vi "PWM Servo RT.vi"() -> ()   [LabVIEW 2012]
uses:
  <vilib>/FPGAPlugInAG/cRIO-9074/niLvFpga_Open_cRIO-9074.vi
  <vilib>/rvi/interface/common/dynamic/niFpgaDynamicAddResources.vi
  <vilib>/Utility/error.llb/Error Cluster From Error Code.vi
  <vilib>/rvi/errors/niLvFpgaAdjustHostInterfaceError.vi
  <vilib>/FPGAPlugInAG/Dynamic/niLvFpga_Close_Dynamic.vi
  <vilib>/rvi/interface/nirviOpenFPGA/nirviOpenFPGA.xnode
  FPGA Bitfiles/MotorLabAProject_FPGATarget_PositionControl(_vtCICTSoXaE.lvbitx
  PWM Servo FPGA.vi
  <vilib>/rvi/interface/nirviReadWriteControl/nirviReadWriteControl.xnode
  <vilib>/rvi/interface/nirviCloseFPGA/nirviCloseFPGA.xnode
  NiFpgaLv.dll
  <vilib>/rvi/interface/Simulation/niFpgaSimulationCallBeginRW.vi
panel:
  out "Drive Status":T1(ring)
  in  "Current Limit (Amps)":dbl
  out "Current Chart":T2(graph)
  out "Trig AI/Heartbeat":bool
  in  "stop":bool
  out "Position Chart":T3(graph)
  in  "Position Setpoint (deg)":i32(knob) scale=0.0..10.0
  in  "PID Gains":T4
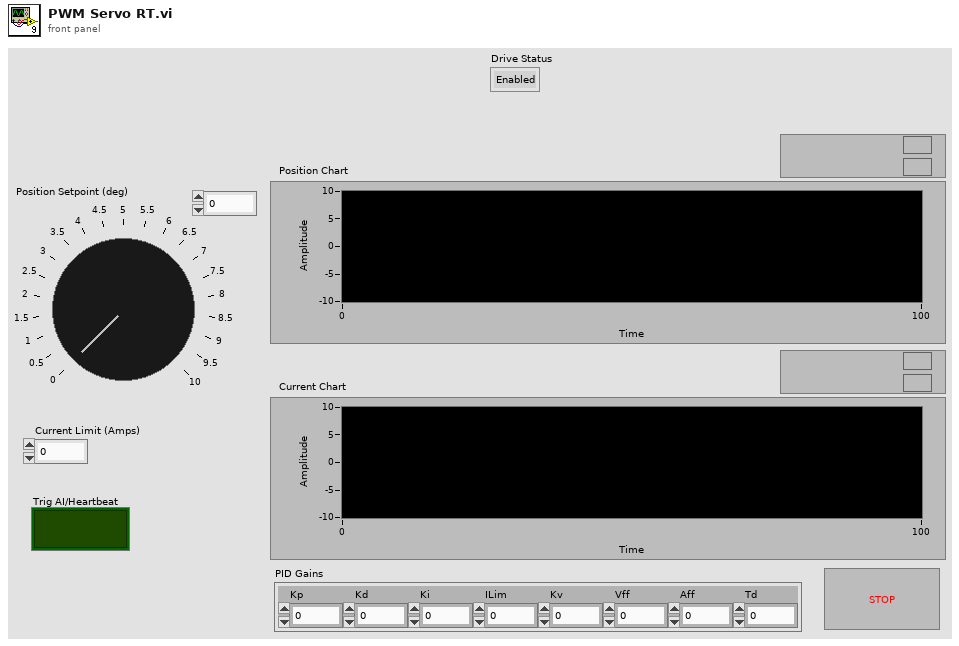
[diagram p1: front panel]
types:
  T1 = enum8{"Enabled", "Disabled", "Disabled by Drive Fault", "Disabled by Temp. Fault", "Disabled by E-Stop", "Unknown"}
  T2 = cluster{"Current Command":i16, "Current Feedback":i16}
  T3 = cluster{"Position Setpoint":i32, "Encoder Position":i32}
  T4 = cluster{"Kp":i16, "Kd":i16, "Ki":i16, "ILim":i16, "Kv":i16, "Vff":i16, "Aff":i16, "Td":i16}
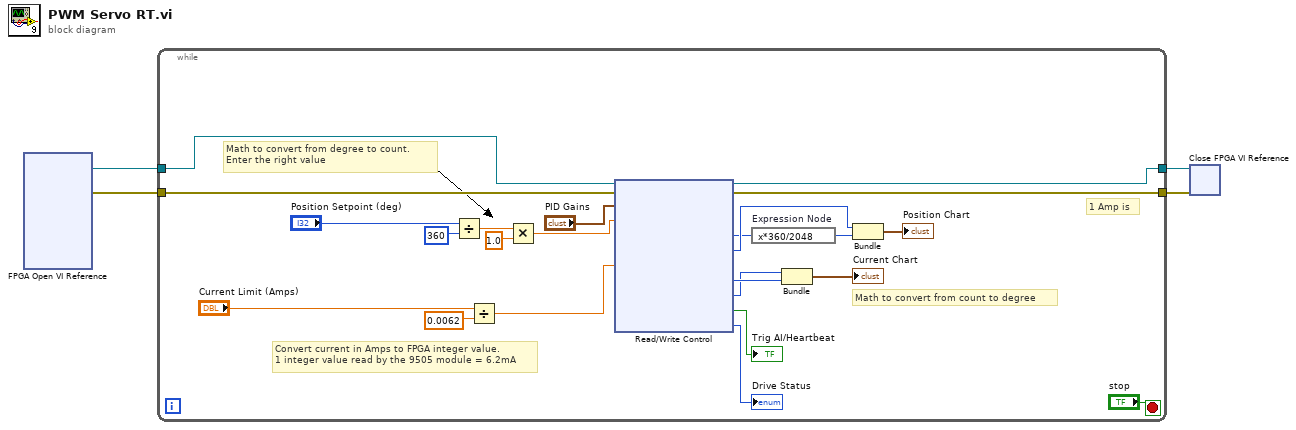
[diagram p0: block diagram]
diagram:
  n1 = xnode "FPGA Open VI Reference"() -> ("FPGA VI Reference Out"=w3:refnum<k20>, "error out"=w4:errorcluster)  [unwired: 2 in]
  n2 = while {
    tunnel: w4 -> [w13]
    tunnel: w3 -> [w14]
    tunnel: [w21] -> w2
    tunnel: [w20] -> w1
    stop <- "stop" stop-if-true
    # "Convert current in Amps to FPGA integer value.\n1 integer value read by the 9505 module = 6.2mA"
    # "1 Amp is"
    # "Math to convert from count to degree"
    # "Math to convert from degree to count.  \nEnter the right value"
    n3 = Divide(x="Position Setpoint (deg)", y=360) -> (x/y=w24:dbl)
    n4 = Divide(x="Current Limit (Amps)", y=0.0062) -> (x/y=w7:dbl)
    n5 = Multiply(x=w24, y=1.0) -> (x*y=w22:dbl)
    n6 = xnode "Read/Write Control"("FPGA VI Reference In"=w14, "error in"=w13, "Position PID Gains"="PID Gains", "Position Setpoint"=w22, "Current Command"=w7) -> ("FPGA VI Reference Out"=w20:refnum<k20>, "error out"=w21:errorcluster, "Encoder Position"=w17:i32, "Position Setpoint"=w19:i32, "Current Feedback"=w11:i16, "Current Command"=w10:i16, "Trig AI"=→"Trig AI/Heartbeat":bool, "Drive Status"=→"Drive Status":T1)
    n7 = expression code="x*360/2048"(w17) -> (w16:i32)
    n8 = Bundle "Bundle"("Current Command"=w10, "Current Feedback"=w11) -> (→"Current Chart":T2)  [unwired: 1 in]
    n9 = Bundle "Bundle"("Position Setpoint"=w19, "Encoder Position"=w16) -> (→"Position Chart":T3)  [unwired: 1 in]
  }
  n10 = xnode "Close FPGA VI Reference"("FPGA VI Reference In"=w1, "error in"=w2) -> ()  [unwired: 1 out]
